vi "PathPlanner_PathConstraints_GetMaxAngularAcceleration.vi"(11 "PathPlannerConstraints":T1={"MaxVelocityMps;"=0.0, "MaxAccelerationMpsSq;"=0.0, "MaxAngularVelRadPsEc;"=0.0, "MaxAngularAccRadPSecSq"=0.0, "Exists"=FALSE, "Unlimited"=FALSE, "NominalVoltageVolts"=12.0}) -> (3 "MaxAngularAccRadPSecSq":dbl)   [LabVIEW 2019, in "PathPlanner24.lvlib"]
doc: "Get max angular acceleration of Path Constraints cluster\n\nInputs:\n - PathConstraint - cluster - The path constraints to query\n\nOutputs:\n - maxAngularAccelerationRpsSq - double - Max angular acceleration (Rad/S^2)"
uses:
  PathPlanner24.lvlib
  TypeDef/PathPlannerPathConstraints.ctl
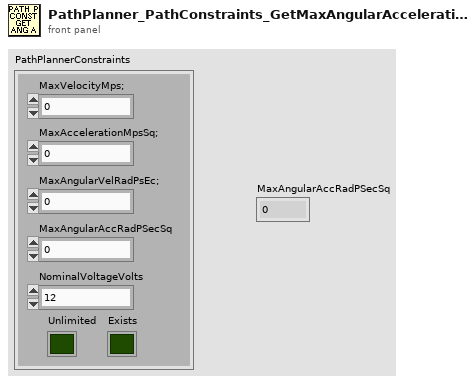
[diagram p1: front panel]
types:
  T1 = typedef "PathPlanner24.lvlib/PathPlannerPathConstraints.ctl" = cluster{"MaxVelocityMps;":dbl, "MaxAccelerationMpsSq;":dbl, "MaxAngularVelRadPsEc;":dbl, "MaxAngularAccRadPSecSq":dbl, "Exists":bool, "Unlimited":bool, "NominalVoltageVolts":dbl}
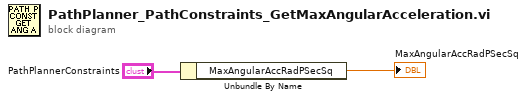
[diagram p0: block diagram]
diagram:
  n1 = Unbundle By Name("PathPlannerConstraints") -> ("MaxAngularAccRadPSecSq"=→"MaxAngularAccRadPSecSq":dbl)
